vi "XYStage_Communication.vi"(8 "error in (no error)":errorcluster, 9 "Command Array":T1(array[cluster])=[[{"Serial Command"="ACCEL", "Expected Reply"="null"}, {"Serial Command"="AALIGN", "Expected Reply"=":A"}, {"Serial Command"="AHOME", "Expected Reply"="null"}, {"Serial Command"="AIJ", "Expected Reply"="null"}, {"Serial Command"="ARRAY", "Expected Reply"="null"}, {"Serial Command"="AZERO", "Expected Reply"="null"}, {"Serial Command"="BACKLASH", "Expected Reply"=":A"}, {"Serial Command"="BCUSTOM", "Expected Reply"="null"}, {"Serial Command"="BENABLE", "Expected Reply"="null"}, {"Serial Command"="BUILD", "Expected Reply"="null"}, {"Serial Command"="CDATE", "Expected Reply"="null"}, {"Serial Command"="CNTS", "Expected Reply"=":A"}, {"Serial Command"="CUSTOMA", "Expected Reply"="null"}, {"Serial Command"="CUSTOMB", "Expected Reply"="null"}, {"Serial Command"="DACK", "Expected Reply"=":A"}, {"Serial Command"="DUMP", "Expected Reply"="null"}, {"Serial Command"="ENSYNC", "Expected Reply"="null"}, {"Serial Command"="EPOLARITY", "Expected Reply"="null"}, {"Serial Command"="ERROR", "Expected Reply"=":A"}, {"Serial Command"="HALT", "Expected Reply"=":A"}, {"Serial Command"="HERE", "Expected Reply"=":A"}, {"Serial Command"="HOME", "Expected Reply"=":A"}, {"Serial Command"="INFO", "Expected Reply"="Ax"}, {"Serial Command"="JOYSTICK", "Expected Reply"=":A"}, {"Serial Command"="JSSPD", "Expected Reply"=":A"}, {"Serial Command"="KD", "Expected Reply"="null"}, {"Serial Command"="KI", "Expected Reply"="null"}, {"Serial Command"="KP", "Expected Reply"="null"}, {"Serial Command"="LCD", "Expected Reply"="null"}, {"Serial Command"="LED", "Expected Reply"="null"}, {"Serial Command"="LLADDR", "Expected Reply"="null"}, {"Serial Command"="LOAD", "Expected Reply"="null"}, {"Serial Command"="MAINTAIN", "Expected Reply"=":A"}, {"Serial Command"="MOTCTRL", "Expected Reply"=":A"}, {"Serial Command"="MOVE", "Expected Reply"=":A"}, {"Serial Command"="MOVREL", "Expected Reply"=":A"}, {"Serial Command"="PCROS", "Expected Reply"=":A"}, {"Serial Command"="PEDAL", "Expected Reply"=":A"}, {"Serial Command"="RBMODE", "Expected Reply"="null"}, {"Serial Command"="RDADC", "Expected Reply"=":A"}, {"Serial Command"="RDSBYTE", "Expected Reply"="null"}, {"Serial Command"="RDSTAT", "Expected Reply"=":A"}, {"Serial Command"="RESET", "Expected Reply"=":A"}, {"Serial Command"="RT", "Expected Reply"=":A"}, {"Serial Command"="RUNAWAY", "Expected Reply"=":A"}, {"Serial Command"="SAVESET", "Expected Reply"=":A"}, {"Serial Command"="SAVEPOS", "Expected Reply"=":A"}, {"Serial Command"="SCAN", "Expected Reply"="null"}, {"Serial Command"="SCANR", "Expected Reply"="null"}, {"Serial Command"="SCANV", "Expected Reply"="null"}, {"Serial Command"="SECURE", "Expected Reply"=":A"}, {"Serial Command"="SETHOME", "Expected Reply"=":A"}, {"Serial Command"="SETLOW", "Expected Reply"=":A"}, {"Serial Command"="SETUP", "Expected Reply"="null"}, {"Serial Command"="SI", "Expected Reply"=":A"}, {"Serial Command"="SPEED", "Expected Reply"=":A"}, {"Serial Command"="SPIN", "Expected Reply"=":A"}, {"Serial Command"="STATUS", "Expected Reply"="N"}, {"Serial Command"="STOPBITS", "Expected Reply"="null"}, {"Serial Command"="TTL", "Expected Reply"="null"}, {"Serial Command"="UM", "Expected Reply"=":A"}, {"Serial Command"="UNITS", "Expected Reply"=":A"}, {"Serial Command"="VB", "Expected Reply"="null"}, {"Serial Command"="VECTOR", "Expected Reply"=":A"}, {"Serial Command"="VERSION", "Expected Reply"=":A"}, {"Serial Command"="WAIT", "Expected Reply"=":A"}, {"Serial Command"="WHERE", "Expected Reply"=":A"}, {"Serial Command"="WHO", "Expected Reply"=":A"}, {"Serial Command"="WRDAC", "Expected Reply"=":A"}, {"Serial Command"="ZERO", "Expected Reply"=":A"}, {"Serial Command"="Z2B", "Expected Reply"=":A"}, {"Serial Command"="ZS", "Expected Reply"=":A"}, {"Serial Command"="OPEN", "Expected Reply"="null"}, {"Serial Command"="CLOSE", "Expected Reply"="null"}, {"Serial Command"="-0.1", "Expected Reply"="null"}, {"Serial Command"="0.1", "Expected Reply"="null"}, {"Serial Command"="75000", "Expected Reply"="null"}], [{"Serial Command"="ACCEL", "Expected Reply"="null"}, {"Serial Command"="AALIGN", "Expected Reply"=":A"}, {"Serial Command"="AHOME", "Expected Reply"="null"}, {"Serial Command"="AIJ", "Expected Reply"="null"}, {"Serial Command"="ARRAY", "Expected Reply"="null"}, {"Serial Command"="AZERO", "Expected Reply"="null"}, {"Serial Command"="BACKLASH", "Expected Reply"=":A"}, {"Serial Command"="BCUSTOM", "Expected Reply"="null"}, {"Serial Command"="BENABLE", "Expected Reply"="null"}, {"Serial Command"="BUILD", "Expected Reply"="null"}, {"Serial Command"="CDATE", "Expected Reply"="null"}, {"Serial Command"="CNTS", "Expected Reply"=":A"}, {"Serial Command"="CUSTOMA", "Expected Reply"="null"}, {"Serial Command"="CUSTOMB", "Expected Reply"="null"}, {"Serial Command"="DACK", "Expected Reply"=":A"}, {"Serial Command"="DUMP", "Expected Reply"="null"}, {"Serial Command"="ENSYNC", "Expected Reply"="null"}, {"Serial Command"="EPOLARITY", "Expected Reply"="null"}, {"Serial Command"="ERROR", "Expected Reply"=":A"}, {"Serial Command"="HALT", "Expected Reply"=":A"}, {"Serial Command"="HERE", "Expected Reply"=":A"}, {"Serial Command"="HOME", "Expected Reply"=":A"}, {"Serial Command"="INFO", "Expected Reply"="Ax"}, {"Serial Command"="JOYSTICK", "Expected Reply"=":A"}, {"Serial Command"="JSSPD", "Expected Reply"=":A"}, {"Serial Command"="KD", "Expected Reply"="null"}, {"Serial Command"="KI", "Expected Reply"="null"}, {"Serial Command"="KP", "Expected Reply"="null"}, {"Serial Command"="LCD", "Expected Reply"="null"}, {"Serial Command"="LED", "Expected Reply"="null"}, {"Serial Command"="LLADDR", "Expected Reply"="null"}, {"Serial Command"="LOAD", "Expected Reply"="null"}, {"Serial Command"="MAINTAIN", "Expected Reply"=":A"}, {"Serial Command"="MOTCTRL", "Expected Reply"=":A"}, {"Serial Command"="MOVE", "Expected Reply"=":A"}, {"Serial Command"="MOVREL", "Expected Reply"=":A"}, {"Serial Command"="PCROS", "Expected Reply"=":A"}, {"Serial Command"="PEDAL", "Expected Reply"=":A"}, {"Serial Command"="RBMODE", "Expected Reply"="null"}, {"Serial Command"="RDADC", "Expected Reply"=":A"}, {"Serial Command"="RDSBYTE", "Expected Reply"="null"}, {"Serial Command"="RDSTAT", "Expected Reply"=":A"}, {"Serial Command"="RESET", "Expected Reply"=":A"}, {"Serial Command"="RT", "Expected Reply"=":A"}, {"Serial Command"="RUNAWAY", "Expected Reply"=":A"}, {"Serial Command"="SAVESET", "Expected Reply"=":A"}, {"Serial Command"="SAVEPOS", "Expected Reply"=":A"}, {"Serial Command"="SCAN", "Expected Reply"="null"}, {"Serial Command"="SCANR", "Expected Reply"="null"}, {"Serial Command"="SCANV", "Expected Reply"="null"}, {"Serial Command"="SECURE", "Expected Reply"=":A"}, {"Serial Command"="SETHOME", "Expected Reply"=":A"}, {"Serial Command"="SETLOW", "Expected Reply"=":A"}, {"Serial Command"="SETUP", "Expected Reply"="null"}, {"Serial Command"="SI", "Expected Reply"=":A"}, {"Serial Command"="SPEED", "Expected Reply"=":A"}, {"Serial Command"="SPIN", "Expected Reply"=":A"}, {"Serial Command"="STATUS", "Expected Reply"="N"}, {"Serial Command"="STOPBITS", "Expected Reply"="null"}, {"Serial Command"="TTL", "Expected Reply"="null"}, {"Serial Command"="UM", "Expected Reply"=":A"}, {"Serial Command"="UNITS", "Expected Reply"=":A"}, {"Serial Command"="VB", "Expected Reply"="null"}, {"Serial Command"="VECTOR", "Expected Reply"=":A"}, {"Serial Command"="VERSION", "Expected Reply"=":A"}, {"Serial Command"="WAIT", "Expected Reply"=":A"}, {"Serial Command"="WHERE", "Expected Reply"=":A"}, {"Serial Command"="WHO", "Expected Reply"=":A"}, {"Serial Command"="WRDAC", "Expected Reply"=":A"}, {"Serial Command"="ZERO", "Expected Reply"=":A"}, {"Serial Command"="Z2B", "Expected Reply"=":A"}, {"Serial Command"="ZS", "Expected Reply"=":A"}, {"Serial Command"="OPEN", "Expected Reply"="null"}, {"Serial Command"="CLOSE", "Expected Reply"="null"}, {"Serial Command"="-0.1", "Expected Reply"="null"}, {"Serial Command"="0.1", "Expected Reply"="null"}, {"Serial Command"="75000", "Expected Reply"="null"}], [{"Serial Command"="ACCEL", "Expected Reply"="null"}, {"Serial Command"="AALIGN", "Expected Reply"=":A"}, {"Serial Command"="AHOME", "Expected Reply"="null"}, {"Serial Command"="AIJ", "Expected Reply"="null"}, {"Serial Command"="ARRAY", "Expected Reply"="null"}, {"Serial Command"="AZERO", "Expected Reply"="null"}, {"Serial Command"="BACKLASH", "Expected Reply"=":A"}, {"Serial Command"="BCUSTOM", "Expected Reply"="null"}, {"Serial Command"="BENABLE", "Expected Reply"="null"}, {"Serial Command"="BUILD", "Expected Reply"="null"}, {"Serial Command"="CDATE", "Expected Reply"="null"}, {"Serial Command"="CNTS", "Expected Reply"=":A"}, {"Serial Command"="CUSTOMA", "Expected Reply"="null"}, {"Serial Command"="CUSTOMB", "Expected Reply"="null"}, {"Serial Command"="DACK", "Expected Reply"=":A"}, {"Serial Command"="DUMP", "Expected Reply"="null"}, {"Serial Command"="ENSYNC", "Expected Reply"="null"}, {"Serial Command"="EPOLARITY", "Expected Reply"="null"}, {"Serial Command"="ERROR", "Expected Reply"=":A"}, {"Serial Command"="HALT", "Expected Reply"=":A"}, {"Serial Command"="HERE", "Expected Reply"=":A"}, {"Serial Command"="HOME", "Expected Reply"=":A"}, {"Serial Command"="INFO", "Expected Reply"="Ax"}, {"Serial Command"="JOYSTICK", "Expected Reply"=":A"}, {"Serial Command"="JSSPD", "Expected Reply"=":A"}, {"Serial Command"="KD", "Expected Reply"="null"}, {"Serial Command"="KI", "Expected Reply"="null"}, {"Serial Command"="KP", "Expected Reply"="null"}, {"Serial Command"="LCD", "Expected Reply"="null"}, {"Serial Command"="LED", "Expected Reply"="null"}, {"Serial Command"="LLADDR", "Expected Reply"="null"}, {"Serial Command"="LOAD", "Expected Reply"="null"}, {"Serial Command"="MAINTAIN", "Expected Reply"=":A"}, {"Serial Command"="MOTCTRL", "Expected Reply"=":A"}, {"Serial Command"="MOVE", "Expected Reply"=":A"}, {"Serial Command"="MOVREL", "Expected Reply"=":A"}, {"Serial Command"="PCROS", "Expected Reply"=":A"}, {"Serial Command"="PEDAL", "Expected Reply"=":A"}, {"Serial Command"="RBMODE", "Expected Reply"="null"}, {"Serial Command"="RDADC", "Expected Reply"=":A"}, {"Serial Command"="RDSBYTE", "Expected Reply"="null"}, {"Serial Command"="RDSTAT", "Expected Reply"=":A"}, {"Serial Command"="RESET", "Expected Reply"=":A"}, {"Serial Command"="RT", "Expected Reply"=":A"}, {"Serial Command"="RUNAWAY", "Expected Reply"=":A"}, {"Serial Command"="SAVESET", "Expected Reply"=":A"}, {"Serial Command"="SAVEPOS", "Expected Reply"=":A"}, {"Serial Command"="SCAN", "Expected Reply"="null"}, {"Serial Command"="SCANR", "Expected Reply"="null"}, {"Serial Command"="SCANV", "Expected Reply"="null"}, {"Serial Command"="SECURE", "Expected Reply"=":A"}, {"Serial Command"="SETHOME", "Expected Reply"=":A"}, {"Serial Command"="SETLOW", "Expected Reply"=":A"}, {"Serial Command"="SETUP", "Expected Reply"="null"}, {"Serial Command"="SI", "Expected Reply"=":A"}, {"Serial Command"="SPEED", "Expected Reply"=":A"}, {"Serial Command"="SPIN", "Expected Reply"=":A"}, {"Serial Command"="STATUS", "Expected Reply"="N"}, {"Serial Command"="STOPBITS", "Expected Reply"="null"}, {"Serial Command"="TTL", "Expected Reply"="null"}, {"Serial Command"="UM", "Expected Reply"=":A"}, {"Serial Command"="UNITS", "Expected Reply"=":A"}, {"Serial Command"="VB", "Expected Reply"="null"}, {"Serial Command"="VECTOR", "Expected Reply"=":A"}, {"Serial Command"="VERSION", "Expected Reply"=":A"}, {"Serial Command"="WAIT", "Expected Reply"=":A"}, {"Serial Command"="WHERE", "Expected Reply"=":A"}, {"Serial Command"="WHO", "Expected Reply"=":A"}, {"Serial Command"="WRDAC", "Expected Reply"=":A"}, {"Serial Command"="ZERO", "Expected Reply"=":A"}, {"Serial Command"="Z2B", "Expected Reply"=":A"}, {"Serial Command"="ZS", "Expected Reply"=":A"}, {"Serial Command"="OPEN", "Expected Reply"="null"}, {"Serial Command"="CLOSE", "Expected Reply"="null"}, {"Serial Command"="-0.1", "Expected Reply"="null"}, {"Serial Command"="0.1", "Expected Reply"="null"}, {"Serial Command"="75000", "Expected Reply"="null"}]], 10 "Command Write and Read":T2={"XY Stage Model"=enum."ASI_MS2000", "Specific Commands"=[], "String Responses"=[], "Numeric Responses"=[], "Commands"=[], "Command Timeout"=1000, "Command Delay (ms)"=200}, 11 "VISA Connection":T5={"Enable termination char"=TRUE, "Termintation Char"=10, "Timeout"=10000, "VISA resource name"="", "Baud Rate"=9600, "Data bits"=8, "Parity"=enum."None", "Stop Bits"=10, "Flow Control"=0, "Mask Array"=[64, 128]} {"Mask Array" items=["Flush Receive Buffer"=16, "Write Transmit Buffer to Device"=32, "Flush Receive Buffer (No I/O)"=64, "Flush Transmit Buffer"=128]; "Flow Control" items=["None", "XON/XOFF", "RTS/CTS", "XON/XOFF & RTS/CTS", "DTR/DSR", "XON/XOFF & DTR/DSR"]; "Stop Bits" items=["1.0"=10, "1.5"=15, "2.0"=20]; "Data bits" min=5 max=8 step=1; "Termintation Char" format="%.0x"}) -> (0 "error out":errorcluster, 2 "Success":bool, 3 "Command Write and Read out":T2)   [LabVIEW 2013]
uses:
  TypeDefs/VISA_Connection.ctl
  <vilib>/Instr/_visa.llb/VISA Flush IO Buffer Mask.ctl
  TypeDefs/Command_Write_Read.ctl
  TypeDefs/XYStage_Model.ctl
  TypeDefs/Stage_Commands.ctl
  <vilib>/Instr/_visa.llb/VISA Configure Serial Port (Instr).vi
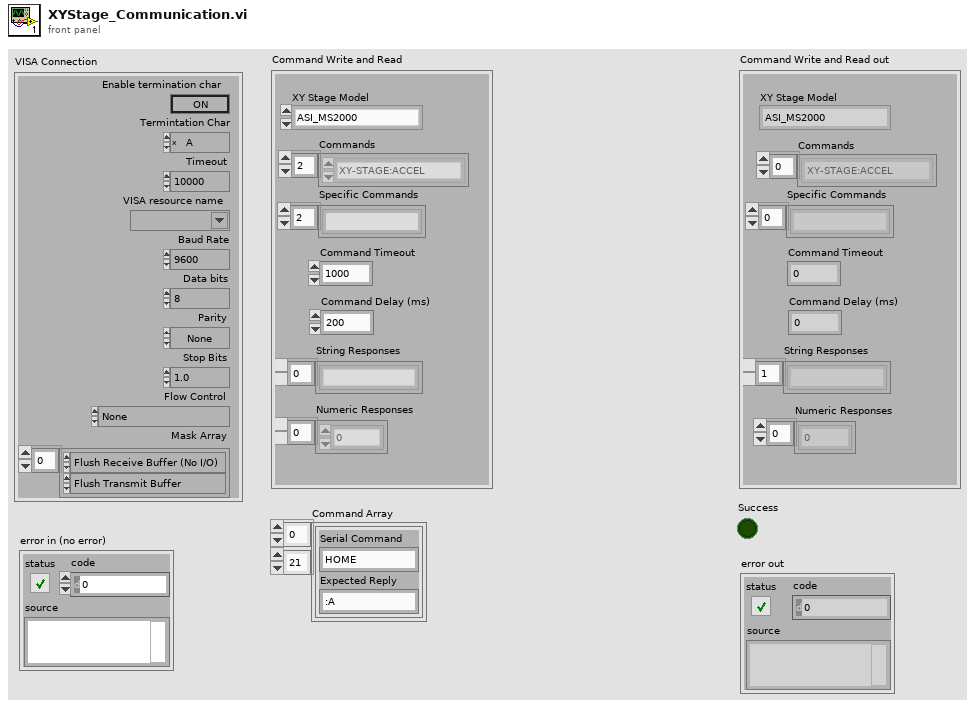
[diagram p1: front panel]
types:
  T1 = cluster{"Serial Command":string, "Expected Reply":string}[][]
  T2 = typedef "Command_Write_Read.ctl" = cluster{"XY Stage Model":T3, "Specific Commands":string[], "String Responses":string[], "Numeric Responses":dbl[], "Commands":T4[], "Command Timeout":i32, "Command Delay (ms)":i32}
  T3 = typedef "XYStage_Model.ctl" = enum16{"ASI_MS2000", "Ludl_Kinetec", "Laurin_Technic"}
  T4 = typedef "Stage_Commands.ctl" = enum16{"XY-STAGE:ACCEL", "XY-STAGE:AALIGN", "XY-STAGE:AHOME", "XY-STAGE:AIJ", "XY-STAGE:ARRAY", "XY-STAGE:AZERO", "XY-STAGE:BACKLASH", "XY-STAGE:BCUSTOM", "XY-STAGE:BENABLE", "XY-STAGE:BUILD", "XY-STAGE:CDATE", "XY-STAGE:CNTS", "XY-STAGE:CUSTOMA", "XY-STAGE:CUSTOMB", "XY-STAGE:DACK", "XY-STAGE:DUMP", "XY-STAGE:ENSYNC", "XY-STAGE:EPOLARITY", "XY-STAGE:ERROR", "XY-STAGE:HALT", "XY-STAGE:HERE", "XY-STAGE:HOME", "XY-STAGE:INFO", "XY-STAGE:JOYSTICK", "XY-STAGE:JSSPD", "XY-STAGE:KD", "XY-STAGE:KI", "XY-STAGE:KP", "XY-STAGE:LCD", "XY-STAGE:LED", "XY-STAGE:LLADDR", "XY-STAGE:LOAD", "XY-STAGE:MAINTAIN", "XY-STAGE:MOTCTRL", "XY-STAGE:MOVE", "XY-STAGE:MOVREL", "XY-STAGE:PCROS", "XY-STAGE:PEDAL", "XY-STAGE:RBMODE", "XY-STAGE:RDADC", "XY-STAGE:RDSBYTE", "XY-STAGE:RDSTAT", "XY-STAGE:RESET", "XY-STAGE:RT", "XY-STAGE:RUNAWAY", "XY-STAGE:SAVESET", "XY-STAGE:SAVEPOS", "XY-STAGE:SCAN", "XY-STAGE:SCANR", "XY-STAGE:SCANV", "XY-STAGE:SECURE", "XY-STAGE:SETHOME", "XY-STAGE:SETLOW", "XY-STAGE:SETUP", "XY-STAGE:SI", "XY-STAGE:SPEED", "XY-STAGE:SPIN", "XY-STAGE:STATUS", "XY-STAGE:STOPBITS", "XY-STAGE:TTL", "XY-STAGE:UM", "XY-STAGE:UNITS", "XY-STAGE:VB", "XY-STAGE:VECTOR", "XY-STAGE:VERSION", "XY-STAGE:WAIT", "XY-STAGE:WHERE", "XY-STAGE:WHO", "XY-STAGE:WRDAC", "XY-STAGE:ZERO", "XY-STAGE:Z2B", "XY-STAGE:ZS", "XY-STAGE:OPEN", "XY-STAGE:CLOSE", "XY-STAGE:XMICRON", "XY-STAGE:YMICRON", "XY-STAGE:SPEED_MAX"}
  T5 = typedef "VISA_Connection.ctl" = cluster{"Enable termination char":bool, "Termintation Char":u8, "Timeout":u32, "VISA resource name":refnum<visa-resource-name>, "Baud Rate":u32, "Data bits":u16, "Parity":enum16{"None", "Odd", "Even", "Mark", "Space"}, "Stop Bits":u16, "Flow Control":u16, "Mask Array":T6[]}
  T6 = typedef "VISA Flush IO Buffer Mask.ctl" = u16
  T7 = cluster{"Serial Command":string, "Expected Reply":string}
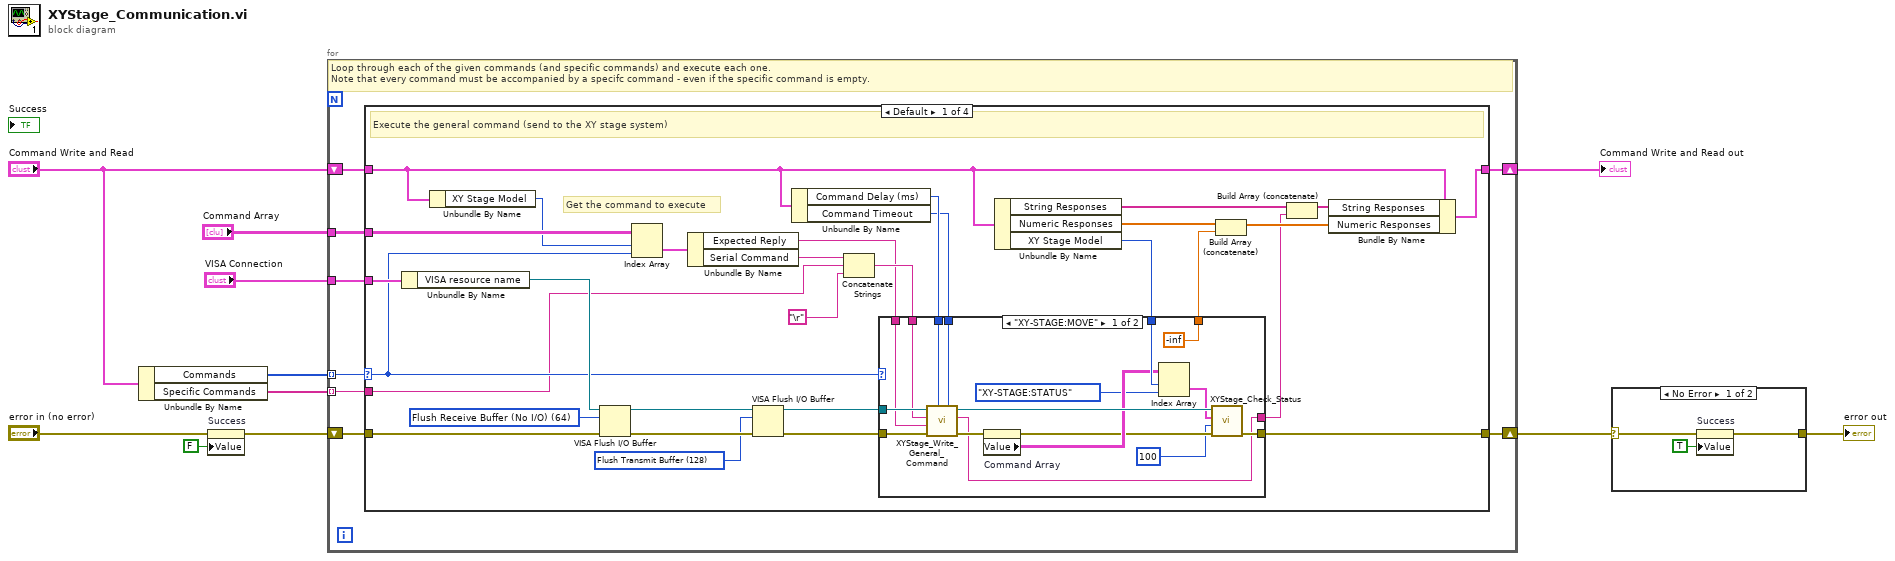
[diagram p0: block diagram]
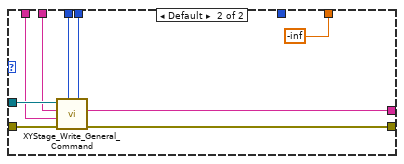
[diagram p3: hidden frame]
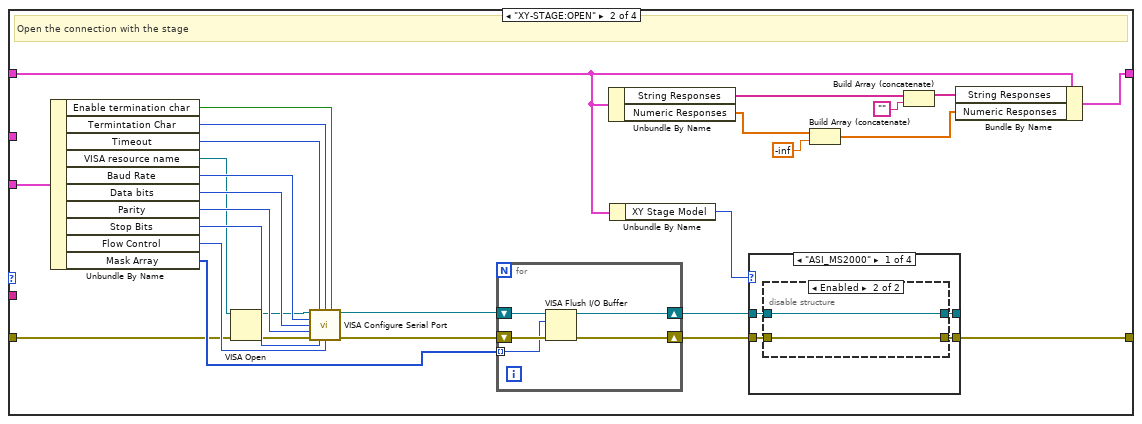
[diagram p4: hidden frame]
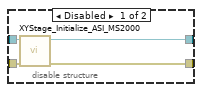
[diagram p5: hidden frame]
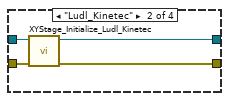
[diagram p6: hidden frame]
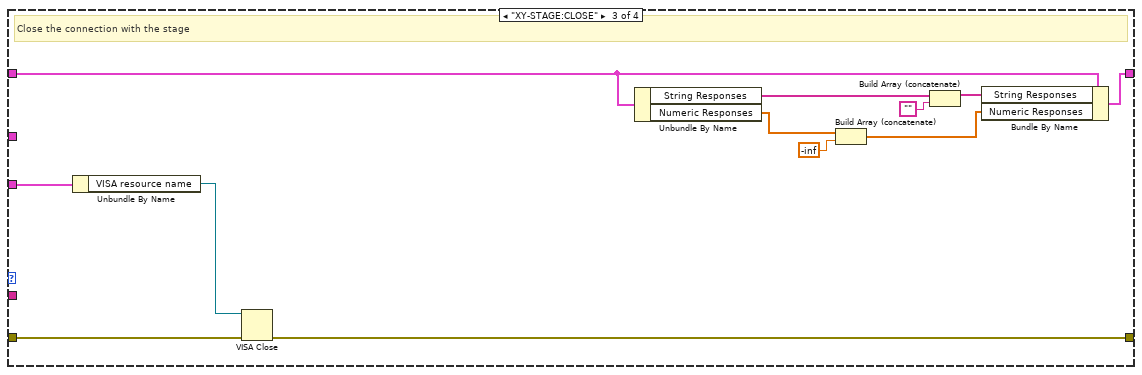
[diagram p9: hidden frame]
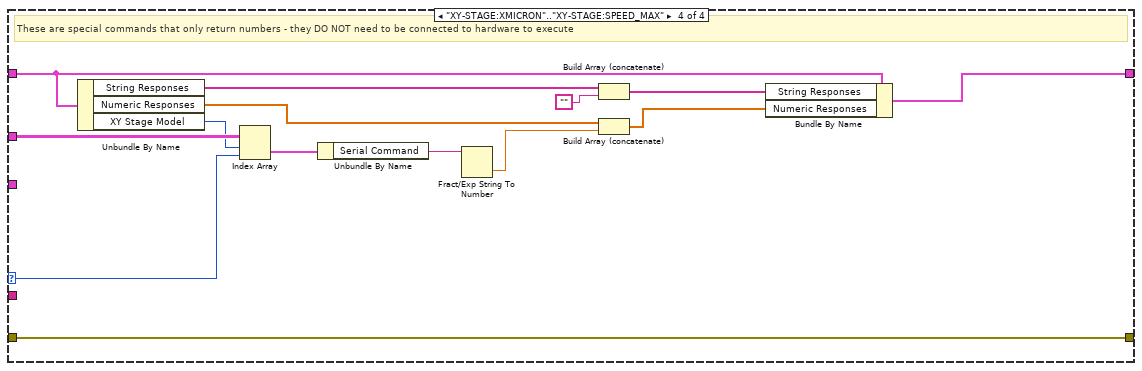
[diagram p10: hidden frame]
diagram:
  n1 = Unbundle By Name("Command Write and Read") -> ("Commands"=w8:T4[], "Specific Commands"=w2:string[])
  n2 = property on="Success" class="Bool (strict)"(error in="error in (no error)", "Value"=FALSE ("Success")) -> (error out=w9:errorcluster)  [unwired: 1 in, 1 out]
  n3 = for {
    tunnel: w8 -> [w12] mode=indexing
    tunnel: "VISA Connection" -> [w18]
    shift-right: [w17] -> w6
    shift-left: w9 -> [w19]
    shift-right: [w16] -> w4
    shift-left: "Command Write and Read" -> [w15]
    tunnel: "Command Array" -> [w14]
    tunnel: w2 -> [w13] mode=indexing
    # "Loop through each of the given commands (and specific commands) and execute each one.\nNote that every command must be accompanied by a specifc command - even if the specific command is empty."
    n4 = case shown="Default" w12 {
      selector: w12 -> [w32 _ _ w149]
      tunnel: w19 -> [w49 w79 w138 w152]
      tunnel: w18 -> [w48 w103 w136 _]
      tunnel: w15 -> [w31 w87 w129 w146]
      tunnel: [w33 w80 w137 w152] -> w17
      tunnel: [w30 w88 w128 w145] -> w16
      tunnel: w14 -> [w42 _ _ w151]
      tunnel: w13 -> [w20 _ _ _]
      frame Default {
        w43 = T6 128 items=["Flush Receive Buffer"=16, "Write Transmit Buffer to Device"=32, "Flush Receive Buffer (No I/O)"=64, "Flush Transmit Buffer"=128] ("Mask")
        w46 = T6 64 items=["Flush Receive Buffer"=16, "Write Transmit Buffer to Device"=32, "Flush Receive Buffer (No I/O)"=64, "Flush Transmit Buffer"=128] ("Mask")
        # "Get the command to execute"
        # "Execute the general command (send to the XY stage system)"
        n5 = Unbundle By Name(w48) -> ("VISA resource name"=w47:refnum<visa-resource-name>)
        n6 = Unbundle By Name(w31) -> ("XY Stage Model"=w41:T3)
        n7 = VISA Flush I/O Buffer(VISA resource name=w47, mask (16)=w46, error in (no error)=w49) -> (VISA resource name out=w44:refnum<visa-resource-name>, error out=w45:errorcluster)
        n8 = Index Array(array=w42, index (row)=w41, index (col)=w32) -> (element=w40:T7)
        n9 = Unbundle By Name(w40) -> ("Expected Reply"=w34:string, "Serial Command"=w39:string)
        n10 = VISA Flush I/O Buffer(VISA resource name=w44, mask (16)=w43, error in (no error)=w45) -> (VISA resource name out=w37:refnum<visa-resource-name>, error out=w38:errorcluster)
        n11 = Unbundle By Name(w31) -> ("Command Delay (ms)"=w36:i32, "Command Timeout"=w23:i32)
        n12 = Concatenate Strings(w39, w20, "\r") -> (w35:string)
        n13 = Unbundle By Name(w31) -> ("String Responses"=w29:string[], "Numeric Responses"=w27:dbl[], "XY Stage Model"=w22:T3)
        n14 = case shown="\"XY-STAGE:MOVE\"" w32 {
          tunnel: w38 -> [w66 w75]
          tunnel: w37 -> [w65 w74]
          tunnel: w36 -> [w62 w73]
          tunnel: w35 -> [w64 w72]
          tunnel: w34 -> [w63 w71]
          tunnel: [w58 w70] -> w33
          tunnel: [-inf -inf] -> w25
          tunnel: [w50 w69] -> w24
          tunnel: w23 -> [w61 w67]
          tunnel: w22 -> [w57 _]
          frame "XY-STAGE:MOVE" {
            n15 = call "XYStage_Write_General_Command.vi"("Timeout"=w61, "Command Delay"=w62, "error in (no error)"=w66, "Expected Reply"=w63, "Command to Execute"=w64, "VISA resource name"=w65) -> ("error out"=w56:errorcluster, "Stage Response"=w50:string, "VISA resource name out"=w59:refnum<visa-resource-name>)  [unwired: 3 in]
            n16 = property on="Command Array" class="Arr (strict)"(error in=w56) -> (error out=w54:errorcluster, "Value"=w55:T1)  [unwired: 1 in, 1 out]
            n17 = Index Array(array=w55, index (row)=w57, index (col)=Stage_Commands."XY-STAGE:STATUS" ("Command Enumerations")) -> (element=w51:T7)
            n18 = call "XYStage_Check_Status.vi"("error in (no error)"=w54, "Number of Status Tries"=100, "Command/Response Cluster"=w51, "VISA resource name"=w59) -> ("error out"=w58:errorcluster)  [unwired: 6 in, 1 out]
          }
          frame Default {
            n19 = call "XYStage_Write_General_Command.vi"("Timeout"=w67, "Command Delay"=w73, "error in (no error)"=w75, "Expected Reply"=w71, "Command to Execute"=w72, "VISA resource name"=w74) -> ("error out"=w70:errorcluster, "Stage Response"=w69:string)  [unwired: 3 in, 1 out]
          }
        }
        n20 = Build Array (concatenate)(w27, w25) -> (w26:dbl[])
        n21 = Build Array (concatenate)(w29, w24) -> (w28:string[])
        n22 = Bundle By Name(cluster=w31, "String Responses"=w28, "Numeric Responses"=w26) -> (w30:T2)
      }
      frame "XY-STAGE:OPEN" {
        # "Open the connection with the stage"
        n23 = Unbundle By Name(w103) -> ("Enable termination char"=w98:bool, "Termintation Char"=w97:u8, "Timeout"=w96:u32, "VISA resource name"=w77:refnum<visa-resource-name>, "Baud Rate"=w95:u32, "Data bits"=w94:u16, "Parity"=w93:enum16{"None", "Odd", "Even", "Mark", "Space"}, "Stop Bits"=w92:u16, "Flow Control"=w91:u16, "Mask Array"=w102:T6[])
        n24 = VISA Open(error in (no error)=w79, VISA resource name=w77) -> (VISA resource name=w76:refnum<visa-resource-name>, error out=w78:errorcluster)  [unwired: 3 in]
        n25 = call-poly "VISA Configure Serial Port"("VISA resource name"=w76, "timeout (10sec)"=w96, "termination char\n(0xA = '\\n' = LF)"=w97, "Enable Termination\nChar (T)"=w98, "baud rate (9600)"=w95, "data bits (8)"=w94, "parity (0:none)"=w93, "error in (no error)"=w78, "stop bits (10: 1 bit)"=w92, "flow control (0:none)"=w91) -> ("VISA resource name out"=w89:refnum<visa-resource-name>, "error out"=w90:errorcluster)  [unwired: 4 in]
        n26 = for {
          shift-right: [w125] -> w99
          shift-left: w90 -> [w126]
          tunnel: w102 -> [w124] mode=indexing
          shift-right: [w123] -> w100
          shift-left: w89 -> [w122]
          n27 = VISA Flush I/O Buffer(VISA resource name=w122, mask (16)=w124, error in (no error)=w126) -> (VISA resource name out=w123:refnum<visa-resource-name>, error out=w125:errorcluster)
        }
        n28 = Unbundle By Name(w87) -> ("String Responses"=w86:string[], "Numeric Responses"=w83:dbl[])
        n29 = Unbundle By Name(w87) -> ("XY Stage Model"=w101:T3)
        n30 = case shown="\"ASI_MS2000\"" w101 {
          tunnel: w100 -> [w106 w116 w118 w120]
          tunnel: w99 -> [w107 w117 w119 w121]
          tunnel: [w105 w115 w119 w121] -> w80
          tunnel: [w104 w114 w118 w120] -> _
          frame "ASI_MS2000" {
            n31 = disable-structure shown="Enabled" {
              disable-tunnel: w107 -> [w111 w112]
              disable-tunnel: w106 -> [w110 w113]
              disable-tunnel: [w109 w112] -> w105
              disable-tunnel: [w108 w113] -> w104
              frame Disabled {
                n32 = call "XYStage_Initialize_ASI_MS2000.vi"("error in (no error)"=w111, "VISA resource name"=w110) -> ("error out"=w109:errorcluster, "VISA resource name out"=w108:refnum<visa-resource-name>)  [unwired: 8 in]
              }
              frame Enabled {
              }
            }
          }
          frame "Ludl_Kinetec" {
            n33 = call "XYStage_Initialize_Ludl_Kinetec.vi"("error in (no error)"=w117, "VISA resource name"=w116) -> ("error out"=w115:errorcluster, "VISA resource name out"=w114:refnum<visa-resource-name>)  [unwired: 8 in]
          }
          frame "Laurin_Technic" {
          }
          frame Default {
          }
        }
        n34 = Build Array (concatenate)(w83, -inf) -> (w81:dbl[])
        n35 = Build Array (concatenate)(w86, "") -> (w85:string[])
        n36 = Bundle By Name(cluster=w87, "String Responses"=w85, "Numeric Responses"=w81) -> (w88:T2)
      }
      frame "XY-STAGE:CLOSE" {
        # "Close the connection with the stage"
        n37 = Unbundle By Name(w136) -> ("VISA resource name"=w135:refnum<visa-resource-name>)
        n38 = VISA Close(VISA resource name=w135, error in (no error)=w138) -> (error out=w137:errorcluster)
        n39 = Unbundle By Name(w129) -> ("String Responses"=w134:string[], "Numeric Responses"=w131:dbl[])
        n40 = Build Array (concatenate)(w131, -inf) -> (w130:dbl[])
        n41 = Build Array (concatenate)(w134, "") -> (w133:string[])
        n42 = Bundle By Name(cluster=w129, "String Responses"=w133, "Numeric Responses"=w130) -> (w128:T2)
      }
      frame "XY-STAGE:XMICRON".."XY-STAGE:SPEED_MAX" {
        # "These are special commands that only return numbers - they DO NOT need to be connected to hardware to execute"
        n43 = Unbundle By Name(w146) -> ("String Responses"=w144:string[], "Numeric Responses"=w141:dbl[], "XY Stage Model"=w150:T3)
        n44 = Index Array(array=w151, index (row)=w150, index (col)=w149) -> (element=w148:T7)
        n45 = Unbundle By Name(w148) -> ("Serial Command"=w147:string)
        n46 = Fract/Exp String To Number(string=w147) -> (number=w142:dbl)  [unwired: 3 in, 1 out]
        n47 = Build Array (concatenate)(w144, "") -> (w143:string[])
        n48 = Build Array (concatenate)(w141, w142) -> (w140:dbl[])
        n49 = Bundle By Name(cluster=w146, "String Responses"=w143, "Numeric Responses"=w140) -> (w145:T2)
      }
    }
  }
  "Command Write and Read out" <- w4
  n50 = case shown="No Error" w6 {
    selector: w6 -> [w154 w156]
    tunnel: [w155 w156] -> w5
    frame No Error {
      n51 = property on="Success" class="Bool (strict)"(error in=w154, "Value"=TRUE ("Success")) -> (error out=w155:errorcluster)  [unwired: 1 in, 1 out]
    }
    frame Error {
    }
  }
  "error out" <- w5
